vi "Close.vi"(8 "Error in (no error)":errorcluster, 11 "VISA resource":refnum<visa-resource-name>) -> (0 "Error out":errorcluster)   [LabVIEW 2010]
doc: "Copyright (c) 2012 Metrolab Technology SA, Plan-les-Ouates, Geneva, Switzerland\nCloses the current session."
uses:
  <vilib>/Instr/_visa.llb/Select Event Type.ctl
panel:
  # "Close"
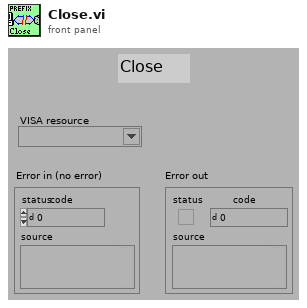
[diagram p1: front panel]
types:
  T1 = typedef "Select Event Type.ctl" = u32
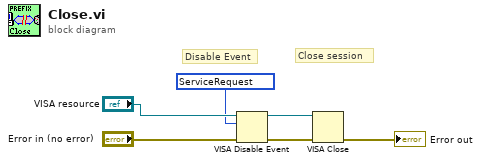
[diagram p0: block diagram]
diagram:
  w1 = T1 1073684491 items=["ServiceRequest"=1073684491, "Trigger"=3221168138, "Clear"=1073684493, "VXI-Signal"=1073684512, "VXI/VME-Interrupt"=3221168161, "VXI/VME-Sysfail"=1073684509, "VXI/VME-Sysreset"=1073684510, "GPIB-CIC"=1073684498, "GPIB-Talk"=1073684499, "GPIB-Listen"=1073684500, "PXI-Interrupt"=1073684514, "Serial-Break"=1073684515, "Serial-TermChar"=1073684516, "Serial-CTS"=1073684521, "Serial-DSR"=1073684522, "Serial-DCD"=1073684524, "Serial-RI"=1073684526, "Serial-Character"=1073684533, "USB-Interrupt"=1073684535, "AllEnabled"=1073709055] ("Event Type")
  # "Disable Event"
  # "Close session"
  n1 = VISA Disable Event(8:"Error in (no error)", 10:w1, 11:"VISA resource") -> (0:w3:errorcluster, 3:w2:refnum<visa-resource-name>)  [unwired: 1 in]
  n2 = VISA Close(VISA resource name=w2, error in (no error)=w3) -> (error out=→"Error out":errorcluster)
